vi "Unflatten Value.vi"(8 "Error In":errorcluster, 10 "Value":string, 11 "2D Int In":refnum<class "2D Int.lvclass">) -> (0 "Error Out":errorcluster, 3 "2D Int Out":refnum<class "2D Int.lvclass">)   [LabVIEW 2020, in "NI_VIAnCFGDataStructure.lvlib" / "2D Int.lvclass"]
doc: "Dynamic dispatch interface for unflattening Tree Data classes from string."
uses:
  <vilib>/addons/analyzer/VIAnCFGDataStructure/Data Types/2D Int/2D Int.lvclass
  <vilib>/addons/analyzer/VIAnCFGDataStructure/Data Types/2D Int/2D Int.lvclass/2D Int.ctl
  <vilib>/addons/analyzer/VIAnCFGDataStructure/Tree Manager/Tree.lvclass
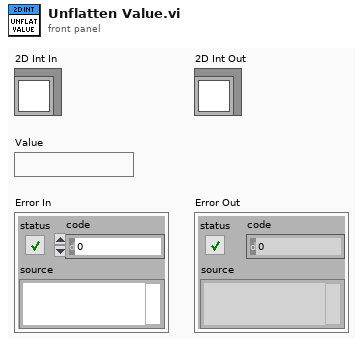
[diagram p1: front panel]
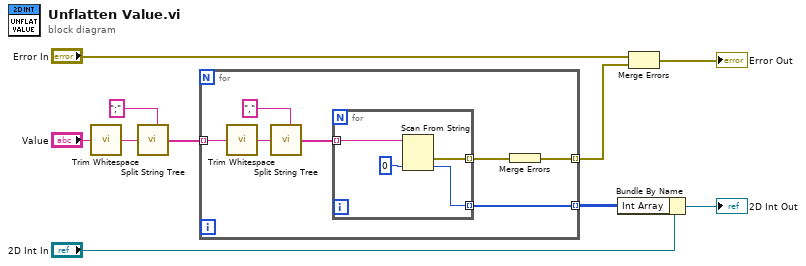
[diagram p0: block diagram]
diagram:
  n1 = call <vilib>:"Trim Whitespace.vi"("string"="Value") -> ("trimmed string"=w1:string)  [unwired: 1 in]
  n2 = call <vilib>:"Split String Tree.vi"("Split Pattern"=";", "Input String"=w1) -> ("Split String"=w9:string[])  [unwired: 5 in]
  n3 = for {
    tunnel: w9 -> [w15] mode=indexing
    tunnel: [w17] -> w8 mode=indexing
    tunnel: [w12] -> w7 mode=indexing
    n4 = call <vilib>:"Trim Whitespace.vi"("string"=w15) -> ("trimmed string"=w11:string)  [unwired: 1 in]
    n5 = call <vilib>:"Split String Tree.vi"("Split Pattern"=",", "Input String"=w11) -> ("Split String"=w14:string[])  [unwired: 5 in]
    n6 = for {
      tunnel: w14 -> [w21] mode=indexing
      tunnel: [w19] -> w17 mode=indexing
      tunnel: [w18] -> w13 mode=indexing
      n7 = Scan From String(input string=w21, default 1=i64 0) -> (error out=w18:errorcluster, output 1=w19:i64)  [unwired: 3 in, 2 out]
    }
    n8 = Merge Errors(w13) -> (w12:errorcluster)
  }
  n9 = Bundle By Name(cluster="2D Int In", "Int Array"=w8) -> (→"2D Int Out":refnum<class "2D Int.lvclass">)
  n10 = Merge Errors("Error In", w7) -> (→"Error Out":errorcluster)
